vi "Measurement UI.vi"() -> ()   [LabVIEW 2021, in "Stepped Frequency Sweep_Audio DAC_UI.lvlib"]
uses:
  Stepped Frequency Sweep_Audio DAC_UI.lvlib
  shared/audio popup ui/Audio Popup UI.lvlib
panel:
  in  "Select Graph":string(combo)="THD+N"
  out "Results graph":cluster{"X array":dbl[], "Y array":dbl[]}[](graph)
  out "Time domain graph":waveform(dbl)[](graph)
  out "Frequency domain graph":cluster{"x0":dbl, "dx":dbl, "magnitude":dbl[]}[](graph)
  in  "settings tab":T1(tab)
  in  "Sweep Profile":string(combo)="Logarithmic" caption="SWEEP PROFILE"
  in  "Sweep Steps":u32=11 caption="SWEEP STEPS"
  in  "Sweep Stop (Hz)":dbl=20000.0 caption="SWEEP STOP" format="%#_6pHz"
  in  "Min settling time (s)":dbl=0.1 caption="MINIMUM SETTLING TIME" format="%#_6ps"
  in  "Min settling cycles":u32 caption="MINIMUM SETTLING CYCLES"
  in  "Min measurement time (s)":dbl=0.1 caption="MINIMUM MEASUREMENT TIME" format="%#_6ps"
  in  "Min measurement cycles":u32 caption="MINIMUM MEASUREMENT CYCLES"
  in  "Sample rate (Hz)":dbl=51200.0 caption="SAMPLE RATE" format="%#_6pHz"
  in  "Acquisition channel":string caption="ACQUISITION CHANNEL"
  in  "Output range (Vpk-pk)":dbl=5.74 caption="OUTPUT RANGE" format="%.3p Vpk-pk"
  in  "Output level units":string(combo)="dBFS" caption="SNR"
  in  "Output level":dbl caption="OUTPUT LEVEL" format="%#_6p"
  in  "Sweep Start (Hz)":dbl=20.0 caption="SWEEP START" format="%#_6pHz"
  in  "Master clock channel":string caption="MASTER CLOCK CHANNEL"
  in  "Digital audio channel":string caption="DIGITAL AUDIO CHANNEL"
  out "digital serial file name":string
  in  "configure digital serial":bool
  in  "Gain units":string(combo)="dB" caption="Gain"
  in  "THD units":string(combo)="dB" caption="THD"
  in  "THD+N units":string(combo)="dB" caption="THD + N"
  in  "SNR units":string(combo)="dB" caption="SNR"
  in  "Band stop (Hz)":dbl=20000.0 caption="BAND STOP" format="%#_6pHz"
  in  "Band start (Hz)":dbl=20.0 caption="BAND START" format="%#_6pHz"
  in  "Weighting filter":string(combo)="A-weighting" caption="WEIGHTING FILTER"
  in  "Lowpass filter":string(combo)="AES17_20kHz" caption="LOWPASS FILTER"
  in  "Highpass filter":string(combo)="AC" caption="HIGHPASS FILTER"
  out "Gain":dbl[](array[numeric]) format="%_6g"
  out "THD":dbl[](array[numeric]) format="%_6g"
  out "THD+N":dbl[](array[numeric]) format="%_6g"
  out "SNR":dbl[](array[numeric]) format="%_6g"
  out "SFDR (dBc)":dbl[](array[numeric]) format="%_6g"
  out "Dynamic range (dB)":dbl[](array[numeric]) format="%_6g"
  out "Phase (deg)":dbl[](array[numeric]) format="%_6g"
  out "Amplitude (dB)":dbl[](array[numeric]) format="%_6g"
  out "Amplitude (V)":dbl[](array[numeric]) format="%_6g"
  out "Frequency (Hz)":dbl[](array[numeric]) format="%_6g"
  out "df":dbl format="%_6g"
  out "f0":dbl format="%_6g"
  out "dt":dbl format="%_6g"
  out "Frequency domain":dbl[](array[numeric]) format="%_6g"
  out "Time domain":dbl[](array[numeric]) format="%_6g"
  out "Channel names":string[](array[string])
  in  "Protocol file":string
  # "Protocol settings"
  # "Generation settings"
  # "Acquisition settings"
  # "Filters"
  # "Units"
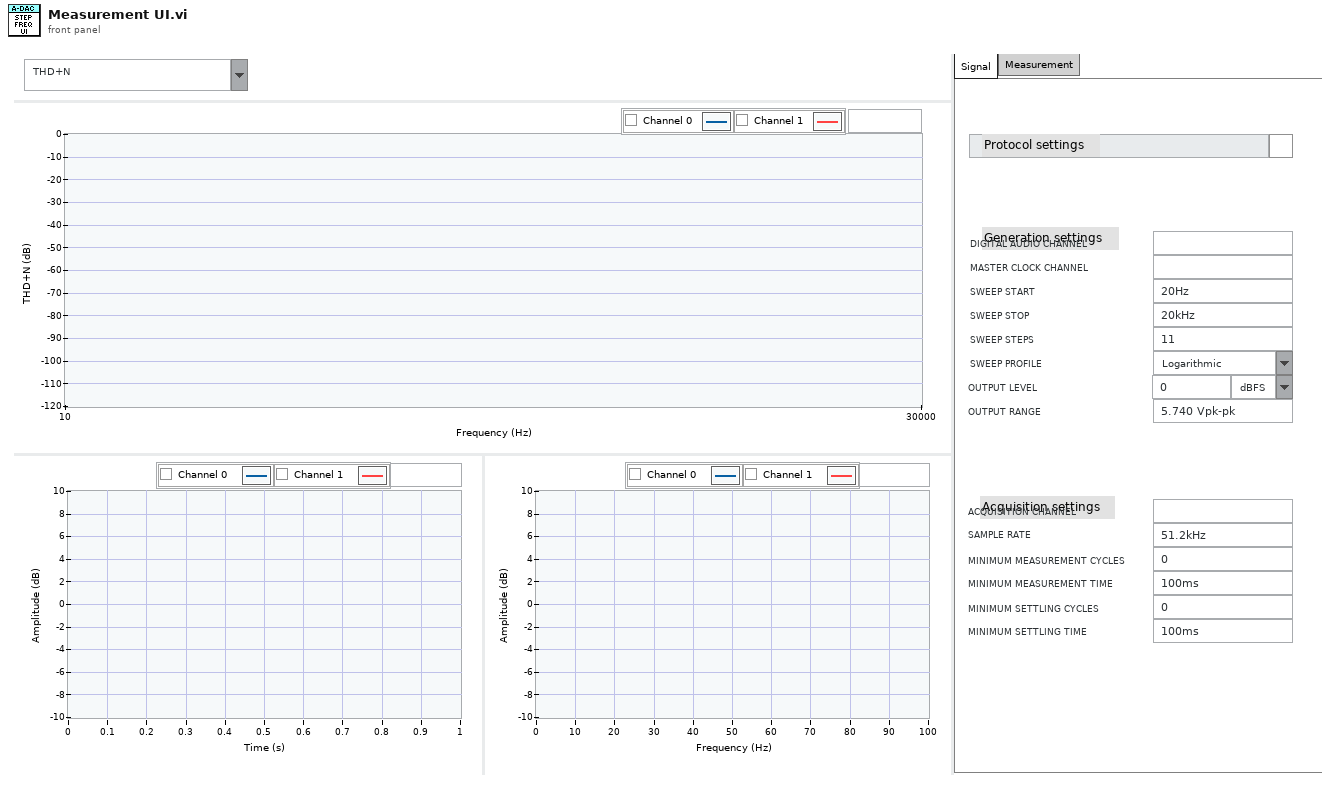
[diagram p1: front panel]
types:
  T1 = enum32{"Signal", "Measurement", "HiddenControls"}
  T2 = typedef "LVBoundsTypeDef.ctl" = cluster{"Width":u32, "Height":u32}
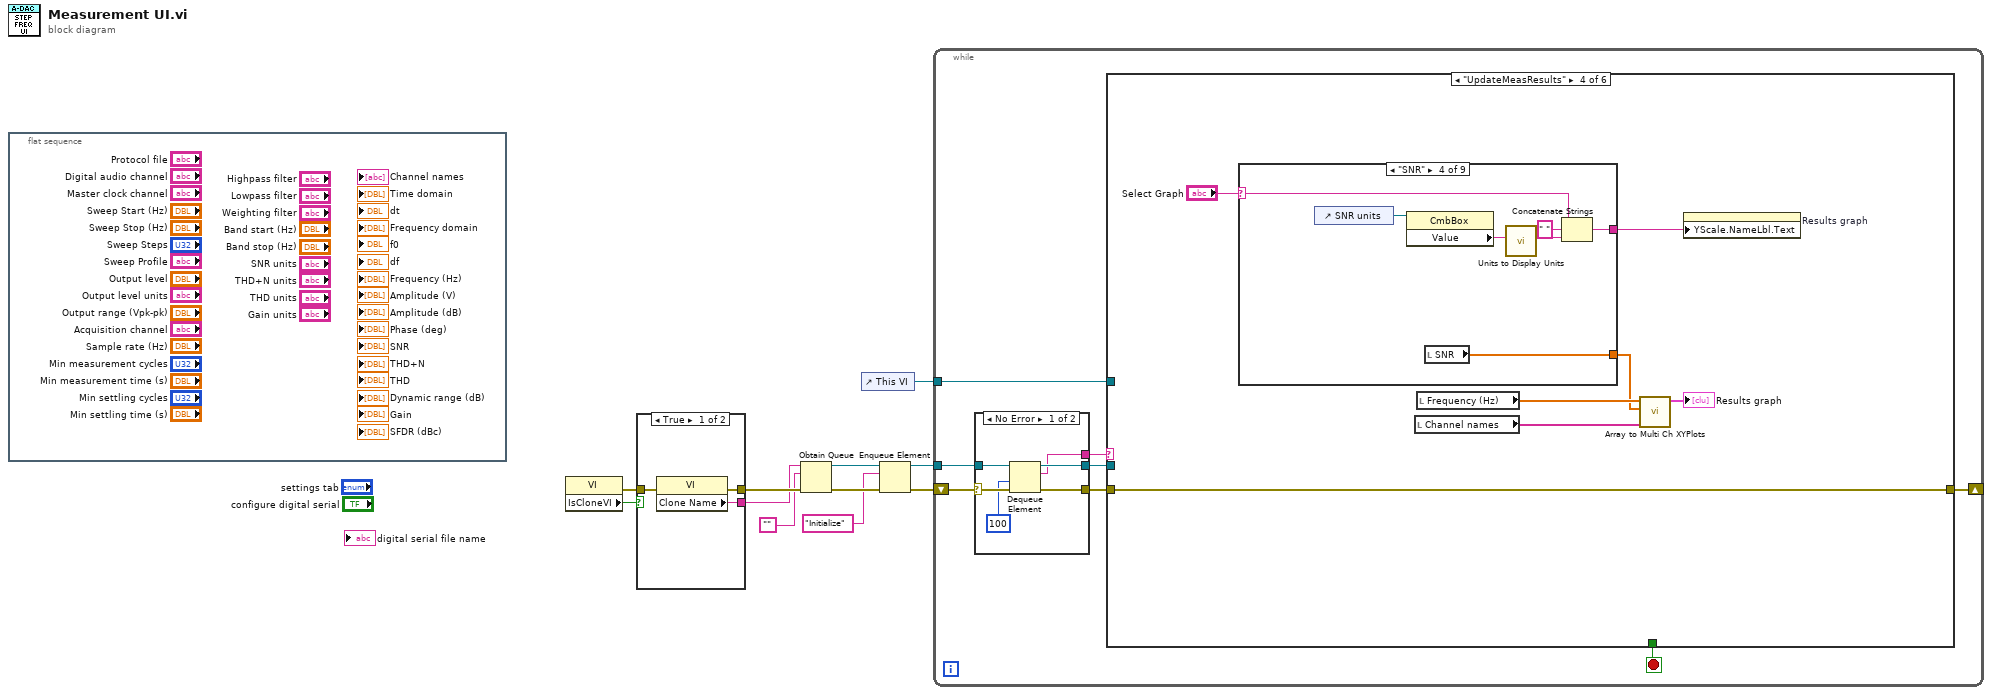
[diagram p0: block diagram]
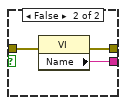
[diagram p2: hidden frame]
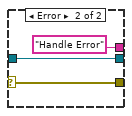
[diagram p3: hidden frame]
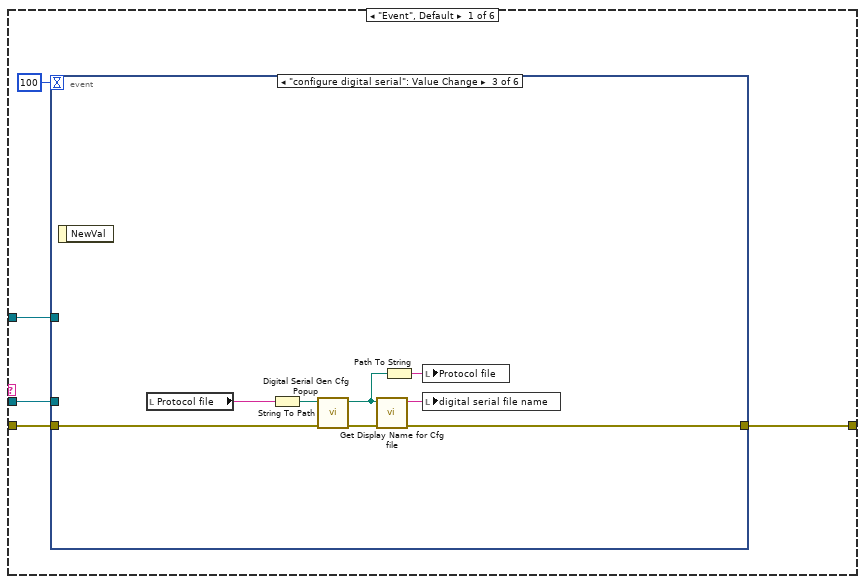
[diagram p4: hidden frame]
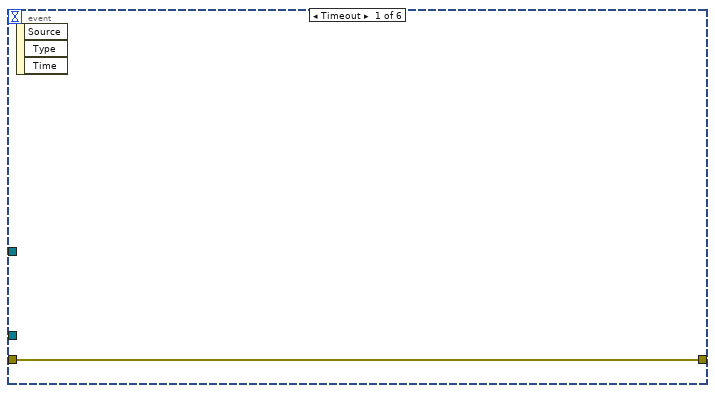
[diagram p5: hidden frame]
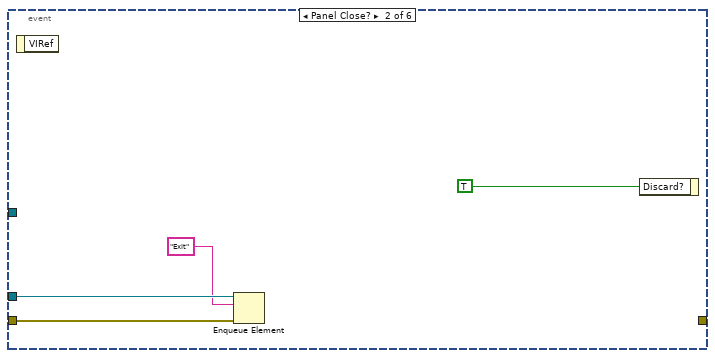
[diagram p6: hidden frame]
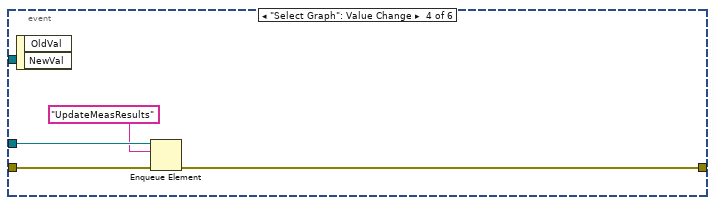
[diagram p7: hidden frame]
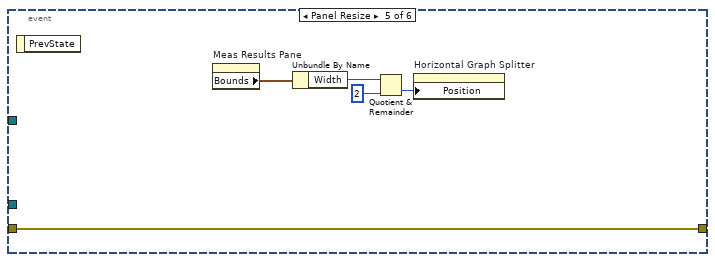
[diagram p8: hidden frame]
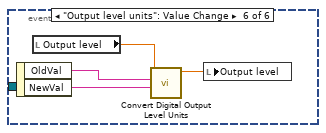
[diagram p9: hidden frame]
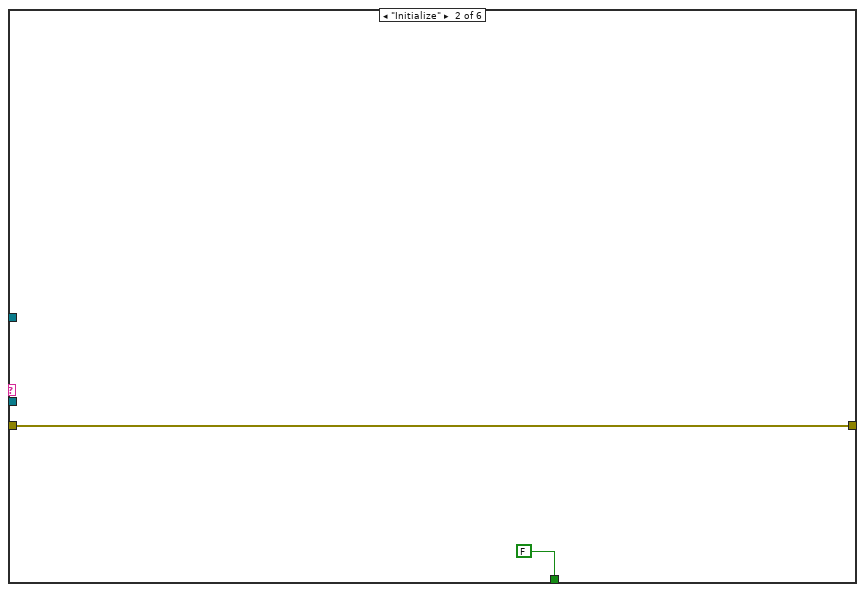
[diagram p10: hidden frame]
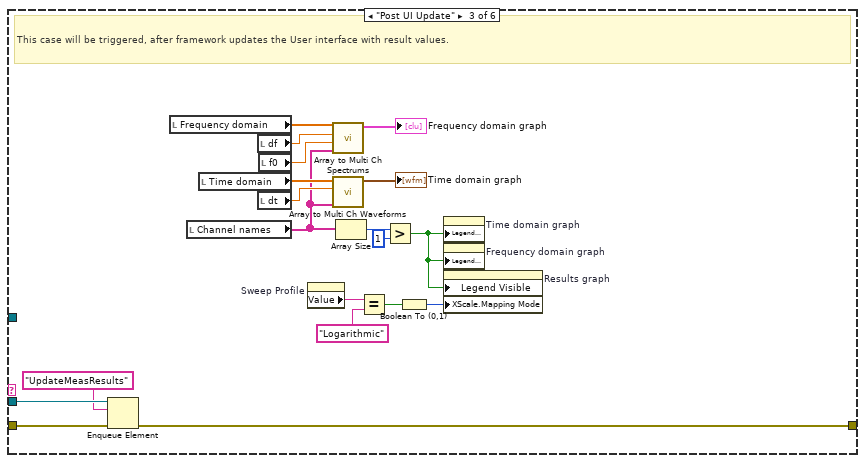
[diagram p11: hidden frame]
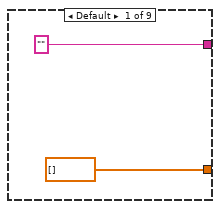
[diagram p12: hidden frame]
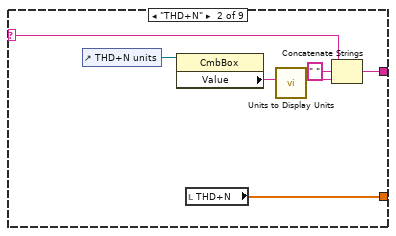
[diagram p13: hidden frame]
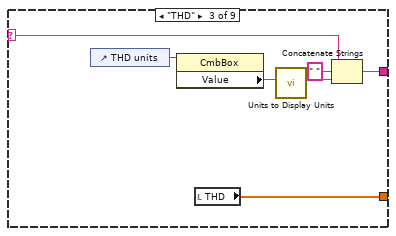
[diagram p14: hidden frame]
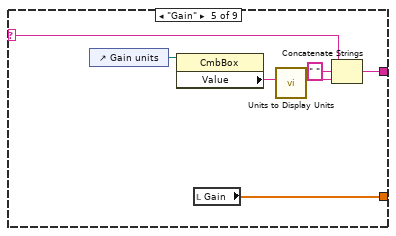
[diagram p15: hidden frame]
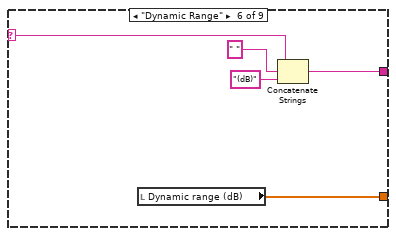
[diagram p16: hidden frame]
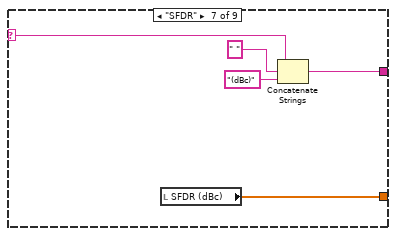
[diagram p17: hidden frame]
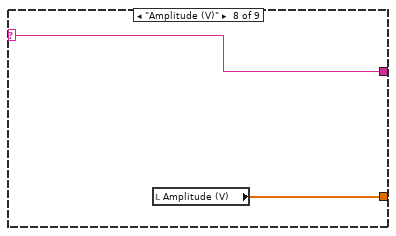
[diagram p18: hidden frame]
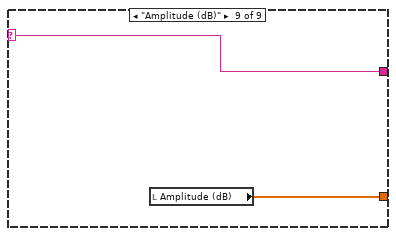
[diagram p19: hidden frame]
diagram:
  n1 = flat-sequence {
    frame #0 {
    }
  }
  n2 = property class="VI"() -> (error out=w2:errorcluster, "IsCloneVI"=w3:bool)  [unwired: 2 in, 1 out]
  n3 = case shown="True" w3 {
    tunnel: [w14 w17] -> w11
    tunnel: [w13 w16] -> w10
    tunnel: w2 -> [w12 w15]
    frame True {
      n4 = property class="VI"(error in=w12) -> (error out=w14:errorcluster, "Clone Name"=w13:string)  [unwired: 1 in, 1 out]
    }
    frame False {
      n5 = property class="VI"(error in=w15) -> (error out=w17:errorcluster, "Name"=w16:string)  [unwired: 1 in, 1 out]
    }
  }
  n6 = Obtain Queue(name (unnamed)=w10, element data type="", error in (no error)=w11) -> (queue out=w7:refnum<queue>, error out=w9:errorcluster)  [unwired: 2 in, 1 out]
  n7 = control-ref of="This VI"() -> (w1:refnum<vi>)
  n8 = Enqueue Element(queue=w7, element="Initialize", error in (no error)=w9) -> (queue out=w6:refnum<queue>, error out=w8:errorcluster)  [unwired: 1 in, 1 out]
  n9 = while {
    shift-right: [w20] -> _
    shift-left: w8 -> [w25]
    tunnel: w6 -> [w23]
    tunnel: w1 -> [w18]
    stop <- w19 stop-if-true
    n10 = case shown="No Error" w25 {
      selector: w25 -> [w31 w34]
      tunnel: [w30 w34] -> w24
      tunnel: w23 -> [w29 w33]
      tunnel: [w28 w33] -> w22
      tunnel: [w27 "Handle Error"] -> w21
      frame No Error {
        n11 = Dequeue Element(queue=w29, timeout in ms (-1)=100, error in (no error)=w31) -> (queue out=w28:refnum<queue>, element=w27:string, error out=w30:errorcluster)  [unwired: 1 out]
      }
      frame Error {
      }
    }
    n12 = case shown="\"UpdateMeasResults\"" w21 {
      tunnel: w24 -> [w38 w67 w73 w93 w138 w145]
      tunnel: w22 -> [w36 _ w75 _ _ w143]
      tunnel: [w39 w67 w74 w93 w138 w140] -> w20
      tunnel: [_ FALSE _ _ _ TRUE] -> w19
      tunnel: w18 -> [w35 _ _ _ _ _]
      frame "Event", Default {
        n13 = event shown="[2] \"configure digital serial\": Value Change" {
          selector: _ -> [_ _ _ _ _ _]
          dyn-events: _ -> [_ _ _ _ _ _]
          timeout: 100 -> [_ _ _ _ _ _]
          tunnel: [w40 _ w51 w53 w61 _] -> w39
          tunnel: w38 -> [w40 w43 w52 w55 w61 _]
          tunnel: w36 -> [_ w42 _ w56 _ _]
          tunnel: w35 -> [_ _ _ _ _ _]
          event Timeout {
            n14 = event-data() -> ()  [unwired: 1 in, 3 out]
          }
          event Panel Close? {
            n15 = event-data() -> ()  [unwired: 1 in, 1 out]
            n16 = Enqueue Element(queue=w42, element="Exit", error in (no error)=w43) -> ()  [unwired: 1 in, 3 out]
            n17 = event-data("Discard?"=TRUE) -> ()  [unwired: 1 in, 1 out]
          }
          event "configure digital serial": Value Change {
            n18 = event-data() -> ()  [unwired: 1 in, 1 out]
            n19 = local read "Protocol file"() -> (w50:string)
            n20 = String To Path(string=w50) -> (path=w49:path)
            n21 = call "Digital Serial Gen Cfg Popup.vi"("error in (no error)"=w52, "config file in"=w49) -> ("error out"=w47:errorcluster, "config file out"=w48:path)  [unwired: 7 in, 1 out]
            n22 = call "Get Display Name for Cfg file.vi"("error in (no error)"=w47, "file path"=w48) -> ("error out"=w51:errorcluster, "display string"=w46:string)  [unwired: 8 in]
            n23 = Path To String(path=w48) -> (string=w45:string)
            n24 = local write "Protocol file"(w45) -> ()
            n25 = local write "digital serial file name"(w46) -> ()
          }
          event "Select Graph": Value Change {
            n26 = event-data() -> ()  [unwired: 1 in, 2 out]
            n27 = Enqueue Element(queue=w56, element="UpdateMeasResults", error in (no error)=w55) -> (error out=w53:errorcluster)  [unwired: 1 in, 2 out]
          }
          event Panel Resize {
            n28 = event-data() -> ()  [unwired: 1 in, 1 out]
            n29 = property on="Meas Results Pane" class="Pane"() -> ("Bounds"=w60:T2)  [unwired: 2 in, 2 out]
            n30 = Unbundle By Name(w60) -> ("Width"=w59:u32)
            n31 = Quotient & Remainder(x=w59, y=u32 2) -> (floor(x/y)=w57:u32)  [unwired: 1 out]
            n32 = property on="Horizontal Graph Splitter" class="Splitter"("Position"=w57) -> ()  [unwired: 2 in, 2 out]
          }
          event "Output level units": Value Change {
            n33 = event-data() -> ("OldVal"=w65:string, "NewVal"=w64:string)  [unwired: 1 in]
            n34 = local read "Output level"() -> (w63:dbl)
            n35 = call "Convert Digital Output Level Units.vi"("New output level units"=w64, "Previous output level units"=w65, "Previous output level"=w63) -> ("New output level"=w62:dbl)  [unwired: 8 in]
            n36 = local write "Output level"(w62) -> ()
          }
        }
      }
      frame "Initialize" {
      }
      frame "Post UI Update" {
        # "This case will be triggered, after framework updates the User interface with result values."
        n37 = Enqueue Element(queue=w75, element="UpdateMeasResults", error in (no error)=w73) -> (error out=w74:errorcluster)  [unwired: 1 in, 2 out]
        n38 = local read "Frequency domain"() -> (w84:dbl[])
        n39 = local read "Channel names"() -> (w76:string[])
        n40 = local read "Time domain"() -> (w86:dbl[])
        n41 = local read "df"() -> (w83:dbl)
        n42 = local read "dt"() -> (w85:dbl)
        n43 = local read "f0"() -> (w82:dbl)
        n44 = property on="Sweep Profile" class="CmbBox"() -> ("Value"=w71:string)  [unwired: 2 in, 2 out]
        n45 = call "Array to Multi Ch Spectrums.vi"("channel names"=w76, "f0"=w82, "df"=w83, "array"=w84) -> ("spectra"=→"Frequency domain graph":cluster{"x0":dbl, "dx":dbl, "magnitude":dbl[]}[])  [unwired: 7 in]
        n46 = call "Array to Multi Ch Waveforms.vi"("channel names"=w76, "dt"=w85, "array"=w86) -> ("waveforms"=→"Time domain graph":waveform(dbl)[])  [unwired: 8 in]
        n47 = Array Size(array=w76) -> (size(s)=w81:i32)
        n48 = Equal?(x=w71, y="Logarithmic") -> (x = y?=w69:bool)
        n49 = Greater?(x=w81, y=1) -> (0:w77:bool)
        n50 = Boolean To (0,1)(Boolean=w69) -> (0, 1=w68:i16)
        n51 = property on="Time domain graph" class="WFGraph (strict)"("Legend Visible"=w77) -> ()  [unwired: 2 in, 2 out]
        n52 = property on="Frequency domain graph" class="WFGraph (strict)"("Legend Visible"=w77) -> ()  [unwired: 2 in, 2 out]
        n53 = property on="Results graph" class="XYGraph (strict)"("Legend Visible"=w77, "XScale.Mapping Mode"=w68) -> ()  [unwired: 2 in, 2 out]
      }
      frame "UpdateMeasResults" {
        n54 = case shown="\"SNR\"" "Select Graph" {
          selector: "Select Graph" -> [_ w100 w107 w114 w121 w126 w131 w134 w136]
          tunnel: [dbl[] [] ("Amplitude (dB)") w102 w109 w116 w123 w128 w133 w135 w137] -> w88
          tunnel: ["" w97 w104 w111 w118 w127 w132 w134 w136] -> w87
          frame Default {
          }
          frame "THD+N" {
            n55 = control-ref of="THD+N units"() -> (w96:refnum<vi>)
            n56 = property class="CmbBox"(reference=w96) -> ("Value"=w101:string)  [unwired: 1 in, 2 out]
            n57 = local read "THD+N"() -> (w102:dbl[])
            n58 = call "Units to Display Units.vi"("Units"=w101) -> ("Display units"=w99:string)  [unwired: 10 in]
            n59 = Concatenate Strings(w100, " " ("string"), w99) -> (w97:string)
          }
          frame "THD" {
            n60 = control-ref of="THD units"() -> (w103:refnum<vi>)
            n61 = property class="CmbBox"(reference=w103) -> ("Value"=w108:string)  [unwired: 1 in, 2 out]
            n62 = local read "THD"() -> (w109:dbl[])
            n63 = call "Units to Display Units.vi"("Units"=w108) -> ("Display units"=w106:string)  [unwired: 10 in]
            n64 = Concatenate Strings(w107, " " ("string"), w106) -> (w104:string)
          }
          frame "SNR" {
            n65 = control-ref of="SNR units"() -> (w110:refnum<vi>)
            n66 = property class="CmbBox"(reference=w110) -> ("Value"=w115:string)  [unwired: 1 in, 2 out]
            n67 = local read "SNR"() -> (w116:dbl[])
            n68 = call "Units to Display Units.vi"("Units"=w115) -> ("Display units"=w113:string)  [unwired: 10 in]
            n69 = Concatenate Strings(w114, " " ("string"), w113) -> (w111:string)
          }
          frame "Gain" {
            n70 = control-ref of="Gain units"() -> (w117:refnum<vi>)
            n71 = property class="CmbBox"(reference=w117) -> ("Value"=w122:string)  [unwired: 1 in, 2 out]
            n72 = local read "Gain"() -> (w123:dbl[])
            n73 = call "Units to Display Units.vi"("Units"=w122) -> ("Display units"=w120:string)  [unwired: 10 in]
            n74 = Concatenate Strings(w121, " " ("string"), w120) -> (w118:string)
          }
          frame "Dynamic Range" {
            n75 = local read "Dynamic range (dB)"() -> (w128:dbl[])
            n76 = Concatenate Strings(w126, " " ("string"), "(dB)" ("string")) -> (w127:string)
          }
          frame "SFDR" {
            n77 = local read "SFDR (dBc)"() -> (w133:dbl[])
            n78 = Concatenate Strings(w131, " " ("string"), "(dBc)" ("string")) -> (w132:string)
          }
          frame "Amplitude (V)" {
            n79 = local read "Amplitude (V)"() -> (w135:dbl[])
          }
          frame "Amplitude (dB)" {
            n80 = local read "Amplitude (dB)"() -> (w137:dbl[])
          }
        }
        n81 = local read "Channel names"() -> (w90:string[])
        n82 = local read "Frequency (Hz)"() -> (w92:dbl[])
        n83 = call "Array to Multi Ch XYPlots.vi"("channel names"=w90, "Y array"=w88, "X array"=w92) -> ("XY plots"=→"Results graph":cluster{"X array":dbl[], "Y array":dbl[]}[])  [unwired: 8 in]
        n84 = property on="Results graph" class="XYGraph (strict)"("YScale.NameLbl.Text"=w87) -> ()  [unwired: 2 in, 2 out]
      }
      frame "Handle Error" {
      }
      frame "Exit" {
        # "This case is triggered to close the User Interface from framework"
        n85 = Flush Queue(queue=w143, error in (no error)=w145) -> (queue out=w142:refnum<queue>, error out=w141:errorcluster)  [unwired: 1 out]
        n86 = Release Queue(queue=w142, force destroy? (F)=TRUE, error in (no error)=w141) -> (error out=w140:errorcluster)  [unwired: 2 out]
      }
    }
  }
